vi "Laser TestBed.vi"() -> ()   [LabVIEW 2022 SP3]
uses:
  abstract laser driver factory/abstract laser driver factory.lvclass
  Laser View/Laser View.lvclass
  088bbc36-e8ae-4795-84b1-81455833b2c3.vi
  <vilib>/Utility/LVClass/Get LV Class Default Value.vi
  XY Stage/Framework/Read Configs/Read Configs Sections.lvlib
  Laser Controller/Laser Controller.lvclass
panel:
  in  "stop":bool
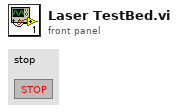
[diagram p1: front panel]
types:
  T1 = typedef "Read Configs Sections.lvlib/Section Data.ctl" = cluster{"Path":path, "Section":string}
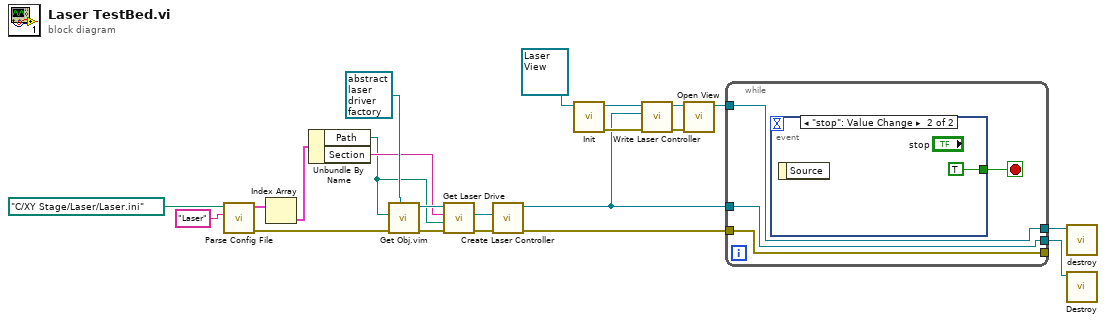
[diagram p0: block diagram]
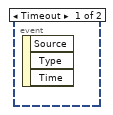
[diagram p2: hidden frame]
diagram:
  n1 = call "Parse Config File.vi"("Section"="Laser", "Config Path"=path "C:/XY Stage/Laser/Laser.ini") -> ("error out"=w18:errorcluster, "Array"=w22:T1[])  [unwired: 8 in]
  n2 = Index Array(array=w22) -> (element=w21:T1)  [unwired: 1 in]
  n3 = Unbundle By Name(w21) -> ("Path"=w13:path, "Section"=w14:string)
  n4 = call "Get Obj.vim"("LabVIEW Object 2"=refnum<class "abstract laser driver factory.lvclass"> refnum ("abstract laser driver factory.lvclass"), "error in (no error)"=w18, "Path"=w13) -> ("error out"=w15:errorcluster, "LabVIEW Object"=w16:refnum<class "abstract laser driver factory.lvclass">)  [unwired: 7 in]
  n5 = call-dynamic "Get Laser Drive.vi"("error in (no error)"=w15, "Path"=w13, "Section"=w14, "abstract laser driver factory in"=w16) -> ("error out"=w11:errorcluster, "Laser Driver.lvclass"=w12:refnum<class "Laser Driver.lvclass">)  [unwired: 6 in]
  n6 = call "Create Laser Controller.vi"("error in (no error)"=w11, "Laser Driver.lvclass"=w12) -> ("error out"=w10:errorcluster, "Laser Controller out"=w1:refnum<class "Laser Controller.lvclass">)  [unwired: 8 in]
  n7 = call-dynamic "Init.vi"("Laser View in"=refnum<class "Laser View.lvclass"> refnum ("Laser View.lvclass")) -> ("error out"=w3:errorcluster, "Laser View out"=w5:refnum<class "Laser View.lvclass">)  [unwired: 9 in]
  n8 = call "Write Laser Controller.vi"("error in (no error)"=w3, "Laser Controller"=w1, "In"=w5) -> ("error out"=w2:errorcluster, "Out"=w4:refnum<class "Laser View.lvclass">)  [unwired: 7 in]
  n9 = call-dynamic "Open View.vi"("error in (no error)"=w2, "base view in"=w4) -> ("base view out"=w8:refnum<class "Laser View.lvclass">)  [unwired: 8 in, 1 out]
  n10 = while {
    tunnel: w1 -> [w26]
    tunnel: [w26] -> w9
    tunnel: w10 -> [w25]
    tunnel: [w25] -> _
    tunnel: w8 -> [w23]
    tunnel: [w23] -> w7
    stop <- w24 stop-if-true
    n11 = event shown="[1] \"stop\": Value Change" {
      selector: _ -> [_ _]
      dyn-events: _ -> [_ _]
      timeout: _ -> [_ _]
      tunnel: [_ TRUE] -> w24
      event Timeout {
        n12 = event-data() -> ()  [unwired: 1 in, 3 out]
      }
      event "stop": Value Change {
        n13 = event-data() -> ()  [unwired: 1 in, 1 out]
      }
    }
  }
  n14 = call-dynamic "destroy.vi"("Laser View in"=w7) -> ()  [unwired: 9 in, 2 out]
  n15 = call "Destroy.vi"("Laser Controller in"=w9) -> ()  [unwired: 9 in, 2 out]
